vi "1 Ch Digital Input.vi"(2 "DI0":refnum<k21>="Chassis1/Mod4/DI0") -> (7 "Packet":u64)   [LabVIEW 2010]
uses:
  <vilib>/eio/EIONode/EIONode.xnode
  <vilib>/rvi/eio/nirviEIOImplementation/nirviEIOImplementation.xnode
  <vilib>/rvi/eio/common/nirviEmuClasses.ctl
  <vilib>/rvi/eio/common/nirviEmuTemplateMethod_noerrors.vi
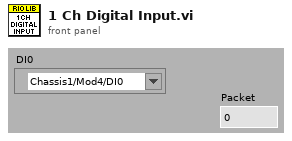
[diagram p1: front panel]
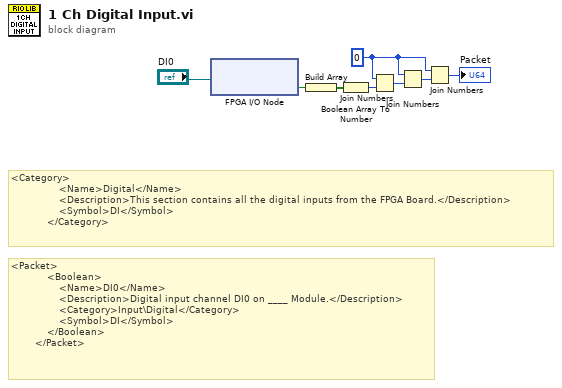
[diagram p0: block diagram]
diagram:
  w2 = u8 0 ("hi")
  # "<Category>\n                <Name>Digital</Name>\n                <Description>This section contains all the digital inputs from the FPGA Board.</Description>\n                <Symbol>DI</Symbol>\n            </Category>"
  # "<Packet>\n            <Boolean>\n                <Name>DI0</Name>\n                <Description>Digital input channel DI0 on ____ Module.</Description>\n                <Category>Input\\Digital</Category>\n                <Symbol>DI</Symbol>\n            </Boolean>\n        </Packet>"
  n1 = xnode "FPGA I/O Node"("FPGA I/O In"="DI0") -> ("I/O Item"=w8:bool)  [unwired: 1 out]
  n2 = Build Array(w8) -> (w7:bool[])
  n3 = Boolean Array To Number(Boolean array=w7) -> (number=w6:u8)
  n4 = Join Numbers(hi=w2, lo=w6) -> ((hi.lo)=w5:u16)
  n5 = Join Numbers(hi=w2, lo=w5) -> ((hi.lo)=w4:u32)
  n6 = Join Numbers(hi=w2, lo=w4) -> ((hi.lo)=→"Packet":u64)
